vi "Open Form.vi"(8 "error in (no error)":errorcluster, 10 "Form Config":refnum<class "Form Configuration.lvclass">, 11 "Form Server in":refnum<class "Form Server.lvclass">) -> (0 "error out":errorcluster, 3 "Form Server out":refnum<class "Form Server.lvclass">)   [LabVIEW 2020, in "Form Server.lvlib" / "Form Server.lvclass"]
uses:
  Form Server.lvclass
  C:/Program Files (x86)/National Instruments/LabVIEW 2020/vi.lib/ActorFramework/Actor/Actor.lvclass
  Form Model/Form Configuration/Form Configuration.lvclass
  Form Model/Form Model.lvclass
  Form Server.lvclass/Form Server.ctl
  <vilib>/ActorFramework/Actor/Actor.lvclass
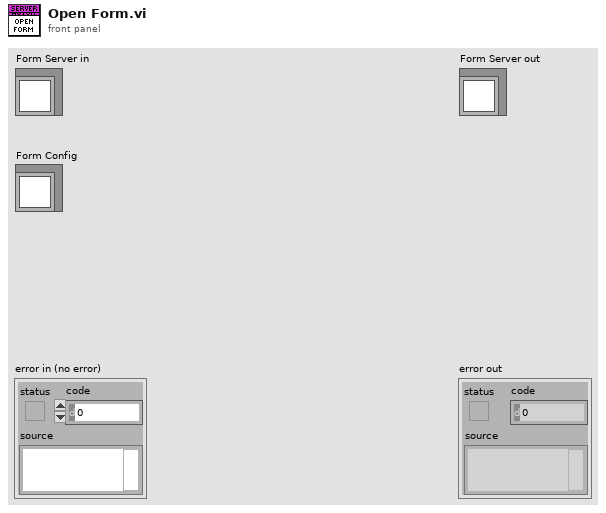
[diagram p1: front panel]
types:
  T1 = typedef "Form Server Interfaces.lvlib/Form ID.ctl" = cluster{"Name":string, "Panel type":string}
  T2 = map{T1, refnum<class "Message Enqueuer.lvclass">}
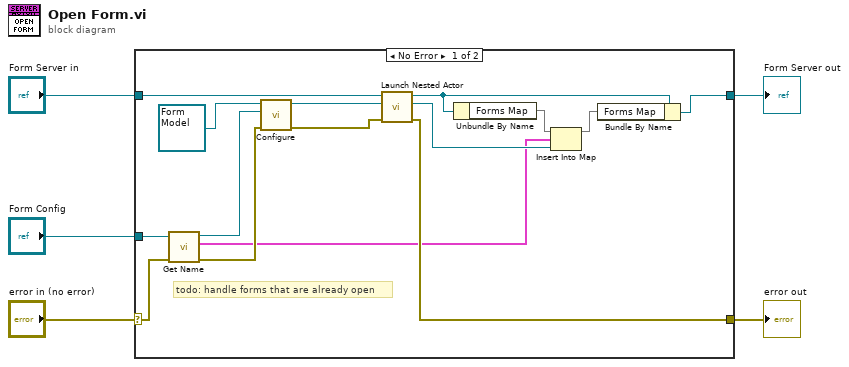
[diagram p0: block diagram]
diagram:
  n1 = case shown="No Error" "error in (no error)" {
    selector: "error in (no error)" -> [w8 w22]
    tunnel: [w19 w22] -> w4
    tunnel: [w13 w21] -> w2
    tunnel: "Form Server in" -> [w20 w21]
    tunnel: "Form Config" -> [w10 _]
    frame No Error {
      # "todo: handle forms that are already open"
      n2 = call-dynamic "Get Name.vi"("error in (no error)"=w8, "Form Configuration in"=w10) -> ("error out"=w7:errorcluster, "Form ID"=w6:T1, "Form Configuration out"=w9:refnum<class "Form Configuration.lvclass">)  [unwired: 7 in]
      n3 = call "Configure.vi"("error in (no error)"=w7, "Configuration"=w9, "Form Model in"=refnum<class "Form Model.lvclass"> refnum ("Form Model.lvlib:Form Model.lvclass")) -> ("error out"=w16:errorcluster, "Form Model out"=w17:refnum<class "Form Model.lvclass">)  [unwired: 7 in]
      n4 = call <vilib>:"Launch Nested Actor.vi"("error in (no error)"=w16, "Nested Actor"=w17, "Caller Actor in"=w20) -> ("error out"=w19:errorcluster, "Nested Actor's Enqueuer"=w11:refnum<class "Message Enqueuer.lvclass">, "Caller Actor out"=w14:refnum<class "Form Server.lvclass">)  [unwired: 6 in]
      n5 = Unbundle By Name(w14) -> ("Forms Map"=w15:T2)
      n6 = Insert Into Map(map in=w15, key=w6, value=w11) -> (map out=w12:T2)  [unwired: 2 out]
      n7 = Bundle By Name(cluster=w14, "Forms Map"=w12) -> (w13:refnum<class "Form Server.lvclass">)
    }
    frame Error {
    }
  }
  "error out" <- w4
  "Form Server out" <- w2
